vi "DAQ_SaveConfig.vi"(8 "error in (no error)":errorcluster, 11 "Message Enqueuer":refnum<class "Message Enqueuer.lvclass">) -> (0 "error out":errorcluster)   [LabVIEW 2025, in "DAQ_API.lvlib"]
uses:
  DAQ_API.lvlib
  DAQ_Module/DAQ_Module/DAQ_Module Messages/SaveConfig Msg/SaveConfig Msg.lvclass
  <vilib>/ActorFramework/Message Enqueuer/Message Enqueuer.lvclass
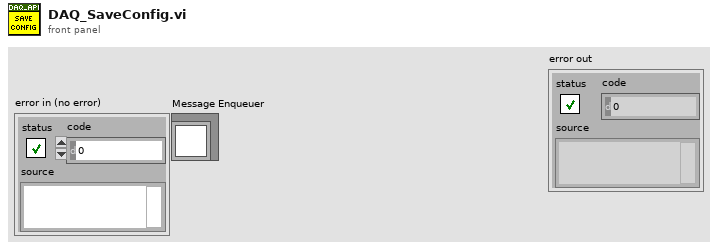
[diagram p1: front panel]
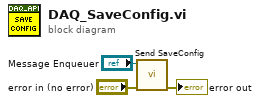
[diagram p0: block diagram]
diagram:
  n1 = call "Send SaveConfig.vi"("error in (no error)"="error in (no error)", "Message Enqueuer"="Message Enqueuer") -> ("error out"=→"error out":errorcluster)  [unwired: 8 in, 1 out]
